vi "Digital Register Analyze.vi"(8 "Published Data Id":string="BoolValid", 9 "Capture Data":u32[](array[numeric]), 10 "Pin Names":string[](array[string]), 11 "Semiconductor Module Context":T1) -> (0 "error out":errorcluster, 2 "Regester":dbl)   [LabVIEW 2014]
uses:
  <vilib>/NI_TestStand_SemiconductorModule/NI_TestStand_Semiconductor_Module.lvlibp/PinMap/General/SemiconductorModuleContext.ctl
  <vilib>/NI_TestStand_SemiconductorModule/NI_TestStand_Semiconductor_Module.lvlibp/PinMap/Digital Pattern/PinsToNIDigitalPatternSessions.vi
  <vilib>/NI_TestStand_SemiconductorModule/NI_TestStand_Semiconductor_Module.lvlibp/PinMap/General/Publish/PublishDataDoubleFunctionalTest.vi
  <vilib>/NI_TestStand_SemiconductorModule/NI_TestStand_Semiconductor_Module.lvlibp
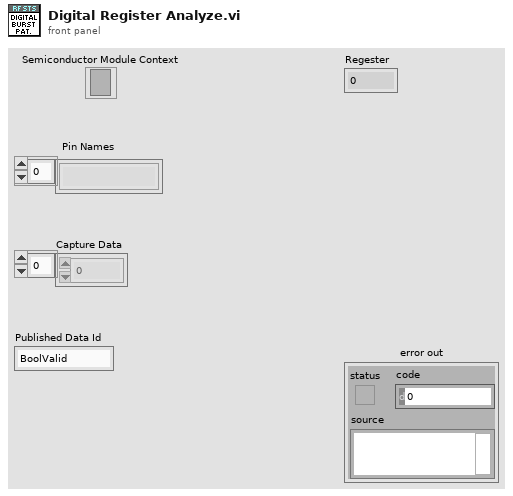
[diagram p1: front panel]
types:
  T1 = typedef "NI_TestStand_Semiconductor_Module.lvlibp/SemiconductorModuleContext.ctl" = refnum<k7>
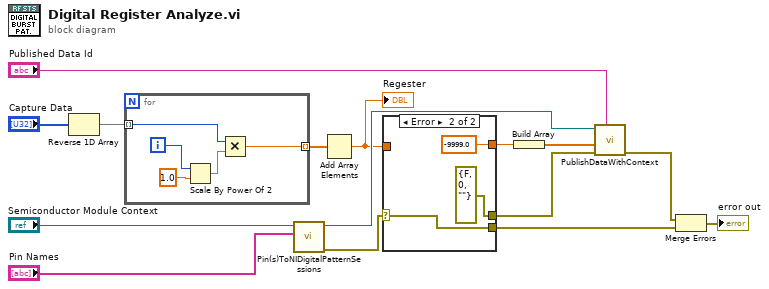
[diagram p0: block diagram]
diagram:
  n1 = Reverse 1D Array(array="Capture Data") -> (reversed array=w1:u32[])
  n2 = for {
    tunnel: w1 -> [w20] mode=indexing
    tunnel: [w17] -> w11 mode=indexing
    i -> [w16]
    n3 = Scale By Power Of 2(n=w16, x=1.0) -> (x*2^n=w18:dbl)
    n4 = Multiply(x=w20, y=w18) -> (x*y=w17:dbl)
  }
  n5 = call-poly <vilib>:"Pin(s)ToNIDigitalPatternSessions.vi"("Pins"="Pin Names", "Semiconductor Module Context"="Semiconductor Module Context") -> ("error out"=w10:errorcluster, "Semiconductor Module Context Out"=w12:T1)  [unwired: 4 in, 4 out]
  n6 = Add Array Elements(numeric array=w11) -> (sum=w6:dbl)
  "Regester" <- w6
  n7 = case shown="Error" w10 {
    selector: w10 -> [w21 w23]
    tunnel: [w21 errorcluster {"status"=FALSE, "code"=0, "source"=""} ("error IO")] -> w9
    tunnel: w6 -> [w22 _]
    tunnel: [w22 -9999.0] -> w8
    tunnel: [w21 w23] -> w4
    frame No Error {
    }
    frame Error {
    }
  }
  n8 = Build Array(w8) -> (w7:dbl[])
  n9 = call-poly <vilib>:"PublishDataWithContext.vi"("Published Data Id"="Published Data Id", "error in (no error)"=w9, "Data In"=w7, "Semiconductor Module Context"=w12) -> ("error out"=w5:errorcluster)  [unwired: 6 in, 1 out]
  n10 = Merge Errors(w5, w4) -> (→"error out":errorcluster)
